vi "Create Events.vi"(8 "error in (no error)":errorcluster) -> (0 "error out":errorcluster, 3 "Event Registration Refnum":refnum<event-registration>)   [LabVIEW 2023]
uses:
  Modules/Controller/Controller.lvlib
  Modules/Template/Template.lvlib
  Controls/FGV Event State.ctl
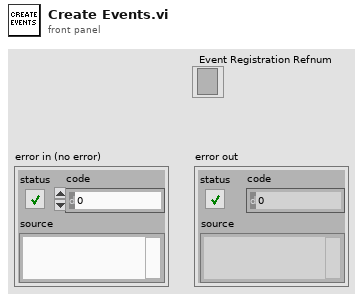
[diagram p1: front panel]
types:
  T1 = typedef "FGV Event State.ctl" = enum16{"Get", "Set"}
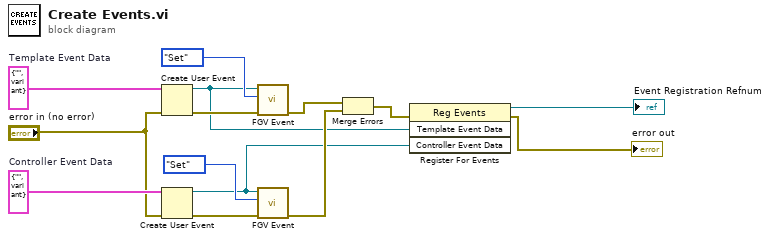
[diagram p0: block diagram]
diagram:
  w13 = cluster{"Event":string, "Data":variant} {"Event"="", "Data"=variant}  # Controller Event Data
  w14 = cluster{"Event":string, "Data":variant} {"Event"="", "Data"=variant}  # Template Event Data
  n1 = Create User Event(user event datatype=w14, error in="error in (no error)") -> (user event=w4:refnum<user-event>, error out=w11:errorcluster)
  n2 = Create User Event(user event datatype=w13, error in="error in (no error)") -> (user event=w3:refnum<user-event>, error out=w10:errorcluster)
  n3 = call "FGV Event.vi"("error in (no error)"=w11, "FGV Event State"=FGV_Event_State."Set", "user event in"=w4) -> ("error out"=w7:errorcluster)  [unwired: 7 in, 1 out]
  n4 = call "FGV Event.vi"("error in (no error)"=w10, "FGV Event State"=FGV_Event_State."Set", "user event in"=w3) -> ("error out"=w6:errorcluster)  [unwired: 7 in, 1 out]
  n5 = Merge Errors(w7, w6) -> (w5:errorcluster)
  n6 = register-events(error in=w5, w4, w3) -> (reference out=→"Event Registration Refnum":refnum<event-registration>, error out=→"error out":errorcluster)  [unwired: 1 in]
